vi "SystemLink_Read.vi"(11 "Thingworx":T1(xcontrol)) -> (1 "number":dbl, 2 "value":string)   [LabVIEW 2019]
uses:
  _Subs/SL_XControl.xctl
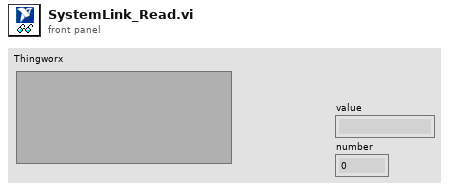
[diagram p1: front panel]
types:
  T1 = cluster{"Tag":string, "Type":string, "Data":string}
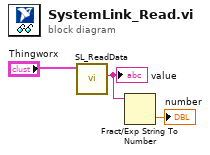
[diagram p0: block diagram]
diagram:
  n1 = call "SL_ReadData.vi"("Tag"="Thingworx") -> ("value"=w3:string)  [unwired: 10 in]
  "value" <- w3
  n2 = Fract/Exp String To Number(string=w3) -> (number=→"number":dbl)  [unwired: 3 in, 1 out]
